vi "CRC-16-CCITT-0xFFFF.vi"(0 "CRC In":u16 format="%.0x", 5 "Reset":bool, 7 "Data":u8 format="%.0x", 11 "error in (no error)":errorcluster) -> (4 "CRC":u16 format="%.0x", 15 "error out":errorcluster)   [LabVIEW 2013]
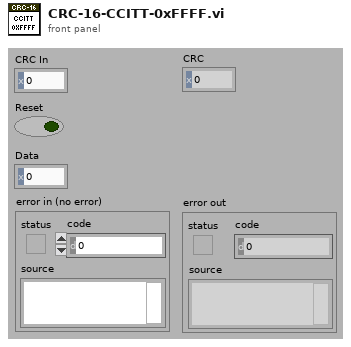
[diagram p1: front panel]
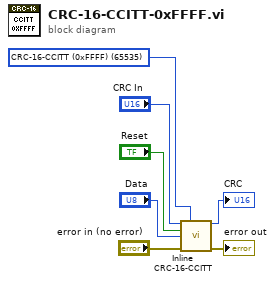
[diagram p0: block diagram]
diagram:
  w5 = u16 65535 items=["CRC-16-CCITT (0x1D0F)"=7439, "CRC-16-CCITT (0xFFFF)"=65535, "CRC-16-CCITT (XModem)"=0] ("CRC-CCITT Type")
  n1 = call "Inline CRC-16-CCITT.vi"("CRC In"="CRC In", "CRC-CCITT Type"=w5, "Reset"="Reset", "Data"="Data", "error in (no error)"="error in (no error)") -> ("CRC"=→"CRC":u16, "error out"=→"error out":errorcluster)  [unwired: 9 in]
